vi "Begin.vi"() -> (0 "error out":errorcluster)   [LabVIEW 2013]
doc: "Called before other user functions, this VI is expected to open initial I/O refnums, load in file data, and do all program initialization. Notice that the <B>error out</B> terminal is simply used for data flow. Wiring it to other structures or subVIs ensures that this VI runs first."
uses:
  <vilib>/Rock Robotics/SystemInterfaces/DIO/FPGA_DIOPWMChannel.ctl
  <vilib>/Rock Robotics/WPI/SafetyOutput/WPI_SafetyOutputConfigMenu.ctl
  <vilib>/Rock Robotics/WPI/DriverStation/WPI_DriverStationRobotMode2.ctl
  <vilib>/Rock Robotics/WPI/Joystick/WPI_JoystickDeviceEnum.ctl
  <vilib>/Rock Robotics/SystemInterfaces/AI/FPGA_AIChannel.ctl
  <vilib>/Rock Robotics/SystemInterfaces/DIO/FPGA_DIORelayChannel.ctl
  <vilib>/Rock Robotics/SystemInterfaces/DIO/FPGA_DIOChannel.ctl
  <vilib>/Rock Robotics/WPI/Solenoid/WPI_SolenoidChannel.ctl
  Robot Global Data.vi
  <vilib>/Rock Robotics/WPI/RobotDrive/WPI_RobotDriveOpen4MotorWithVictor.vi
  <vilib>/Rock Robotics/WPI/Solenoid/WPI_SolenoidOpenDouble.vi
  Robot Global ref.vi
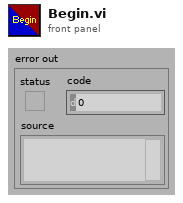
[diagram p1: front panel]
types:
  T1 = typedef "WPI_SolenoidChannel.ctl" = enum8{"Solenoid 1", "Solenoid 2", "Solenoid 3", "Solenoid 4", "Solenoid 5", "Solenoid 6", "Solenoid 7", "Solenoid 8", "Invalid"}
  T2 = typedef "FPGA_DIOChannel.ctl" = enum8{"DIO 1", "DIO 2", "DIO 3", "DIO 4", "DIO 5", "DIO 6", "DIO 7", "DIO 8", "DIO 9", "DIO 10", "DIO 11", "DIO 12", "DIO 13", "DIO 14", "Invalid"}
  T3 = typedef "FPGA_DIORelayChannel.ctl" = enum8{"Relay 1", "Relay 2", "Relay 3", "Relay 4", "Relay 5", "Relay 6", "Relay 7", "Relay 8", "Invalid"}
  T4 = typedef "FPGA_DIOPWMChannel.ctl" = enum8{"PWM 1", "PWM 2", "PWM 3", "PWM 4", "PWM 5", "PWM 6", "PWM 7", "PWM 8", "PWM 9", "PWM 10", "Invalid"}
  T5 = typedef "FPGA_AIChannel.ctl" = enum8{"AI 1", "AI 2", "AI 3", "AI 4", "AI 5", "AI 6", "AI 7", "AI 8", "Invalid"}
  T6 = typedef "WPI_JoystickDeviceEnum.ctl" = enum16{"USB 1", "USB 2", "USB 3", "USB 4", "Kinect 1", "Kinect 2"}
  T7 = typedef "WPI_DriverStationRobotMode2.ctl" = enum16{"Autonomous Disabled", "Autonomous Enabled", "Teleop Disabled", "Teleop Enabled", "Timeout", "Finish", "Test Disabled", "Test Enabled"}
  T8 = typedef "WPI_SafetyOutputConfigMenu.ctl" = enum16{"Enable", "Disable"}
  T9 = typedef "WPI_JoystickDevRef.ctl" = cluster{"Device":T6}
  T10 = typedef "WPI_AnalogChannelDevRef.ctl" = cluster{"DevStatus":errorcluster, "Analog Module":T11, "Analog Channel":T5}
  T11 = typedef "FPGA_TypedefAnalogModule.ctl" = enum16{"Analog Module 1", "Analog Module 2"}
  T12 = typedef "WPI_SolenoidDevRef.ctl" = cluster{"DevStatus":errorcluster, "Solenoid Module":T13, "Forward Solenoid Channel":T1, "Reverse Solenoid Channel":T1}
  T13 = typedef "FPGA_TypedefSolenoidModule.ctl" = enum16{"Solenoid Module 1", "Solenoid Module 2"}
  T14 = typedef "WPI_CompressorDevRef.ctl" = cluster{"DevStatus":errorcluster, "DigitalInputDevRef":T15, "RelayDevRef":T17}
  T15 = typedef "WPI_DigitalInputDevRef.ctl" = cluster{"DevStatus":errorcluster, "DIO Channel":T2, "Digital Module":T16}
  T16 = typedef "FPGA_TypedefDigitalModule.ctl" = enum16{"Digital Module 1", "Digital Module 2"}
  T17 = typedef "WPI_RelayDevRef.ctl" = cluster{"DevStatus":errorcluster, "Relay Channel":T3, "Digital Module":T16, "Relay Direction":T18}
  T18 = typedef "WPI_RelayDirection.ctl" = enum16{"Both directions", "Forward only", "Reverse only"}
  T19 = typedef "WPI_RobotDriveDevRef.ctl" = cluster{"DevStatus":errorcluster, "Motors[]":T20[], "Square Inputs":bool, "Max Output":dbl, "Isochronous":bool}
  T20 = typedef "WPI_MotorControlDeviceRef.ctl" = cluster{"DeviceStatus":errorcluster, "Type":enum16{"PWM", "CAN"}, "PWM":cluster{"Digital Module":T16, "PWM Channel":T4, "DeadBand":T21}, "CAN":cluster{"Device Number":u8, "Control Mode":T22, "Semaphore":T23, "Max Vout":dbl}, "Invert":bool, "TransformRef":T24, "InvTransformRef":T24}
  T21 = typedef "WPI_PWMDeadband.ctl" = cluster{"Name":string, "maxPositivePwm":i32, "minPositivePwm":i32, "centerPwm":i32, "maxNegativePwm":i32, "minNegativePwm":i32, "angularRange":u16}
  T22 = typedef "WPI_CANJaguar_ControlMode.ctl" = enum8{"Percent VBus", "Current", "Speed", "Position", "Voltage"}
  T23 = typedef "Semaphore RefNum" = refnum<k1>
  T24 = typedef "WPI_PWMTransform_ConPane.ctl" = refnum<vi>
  T25 = cluster{"Joysticks":cluster{"OpJoystickRef":T9, "DriveJoystickRef":T9}, "Drive Motors Ref":cluster{"RobotDriveDevRef":T19}, "Ultrasonic":cluster{"AIDeviceRef":T10}, "Comopressor":cluster{"CompressorDevRef":T14}, "Shifters":cluster{"SolenoidDevRef":T12}}
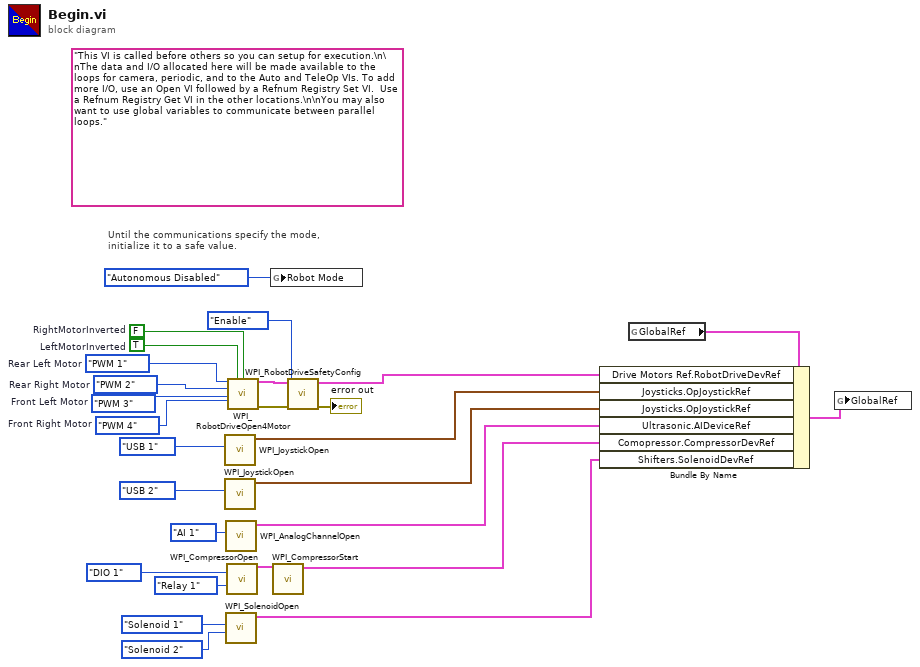
[diagram p0: block diagram]
diagram:
  w8 = FPGA_DIOPWMChannel."PWM 4"  # Front Right Motor
  w9 = FPGA_DIOPWMChannel."PWM 3"  # Front Left Motor
  (unwired) "This VI is called before others so you can setup for execution.\n\nThe data and I/O allocated here will be made available to the loops for camera, periodic, and to the Auto and TeleOp VIs. To add more I/O, use an Open VI followed by a Refnum Registry Set VI.  Use a Refnum Registry Get VI in the other locations.\n\nYou may also want to use global variables to communicate between parallel loops."
  w24 = FPGA_DIOPWMChannel."PWM 2"  # Rear Right Motor
  w25 = FPGA_DIOPWMChannel."PWM 1"  # Rear Left Motor
  w26 = TRUE  # LeftMotorInverted
  w27 = FALSE  # RightMotorInverted
  # "Until the communications specify the mode,\ninitialize it to a safe value."
  n1 = call <vilib>:"WPI_JoystickOpen.vi"("JoystickDevice"=WPI_JoystickDeviceEnum."USB 1") -> ("JoystickDevRef"=w17:T9)  [unwired: 10 in]
  n2 = call <vilib>:"WPI_JoystickOpen.vi"("JoystickDevice"=WPI_JoystickDeviceEnum."USB 2") -> ("JoystickDevRef"=w16:T9)  [unwired: 10 in]
  n3 = call <vilib>:"WPI_AnalogChannelOpen.vi"("Analog Channel"=FPGA_AIChannel."AI 1") -> ("AIDeviceRef"=w10:T10)  [unwired: 9 in, 1 out]
  n4 = call-poly <vilib>:"WPI_SolenoidOpen.vi"("Reverse Solenoid Channel"=WPI_SolenoidChannel."Solenoid 2", "Forward Solenoid Channel"=WPI_SolenoidChannel."Solenoid 1" ("Solenoid Channel")) -> ("SolenoidDevRef"=w2:T12)  [unwired: 8 in, 1 out]
  n5 = call <vilib>:"WPI_CompressorOpen.vi"("Pressure Switch DIO Channel"=FPGA_DIOChannel."DIO 1", "Relay Channel"=FPGA_DIORelayChannel."Relay 1") -> ("CompressorDevRef"=w5:T14)  [unwired: 12 in, 1 out]
  n6 = call-poly <vilib>:"WPI_RobotDriveOpen4Motor.vi"("Rear Left Motor"=w25, "Rear Left Motor Inverted"=w26, "Rear Right Motor Inverted"=w27, "Rear Right Motor"=w24, "Front Left Motor"=w9, "Front Right Motor"=w8) -> ("RobotDriveDevRef"=w15:T19, "error out"=w13:errorcluster)  [unwired: 8 in]
  n7 = global write "Robot Global Data.vi" "Robot Mode"(WPI_DriverStationRobotMode2."Autonomous Disabled" ("Robot Mode")) -> ()
  n8 = call <vilib>:"WPI_CompressorStart.vi"("CompressorDevRef"=w5) -> ("CompressorDevRef"=w4:T14)  [unwired: 9 in, 1 out]
  n9 = call <vilib>:"WPI_RobotDriveSafetyConfig.vi"("error in (no error)"=w13, "mode"=WPI_SafetyOutputConfigMenu."Enable", "RobotDriveDevRef"=w15) -> ("error out"=→"error out":errorcluster, "RobotDriveDevRef"=w14:T19)  [unwired: 7 in]
  n10 = global read "Robot Global ref.vi" "GlobalRef"() -> (w18:T25)
  n11 = Bundle By Name(cluster=w18, "Drive Motors Ref.RobotDriveDevRef"=w14, "Joysticks.OpJoystickRef"=w17, "Joysticks.OpJoystickRef"=w16, "Ultrasonic.AIDeviceRef"=w10, "Comopressor.CompressorDevRef"=w4, "Shifters.SolenoidDevRef"=w2) -> (w19:T25)
  n12 = global write "Robot Global ref.vi" "GlobalRef"(w19) -> ()
